vi "OFBS_test_Classifier.vi"(6 "Test Data":T2, 8 "error in (no error)":errorcluster, 9 "Classifier Session":T1, 10 "Parameters":i32[](array[numeric]), 11 "OFBS class in":refnum<class "OptFreqBandsSearch.lvclass">) -> (0 "error out":errorcluster, 1 "Confusion Matrix":i32[][](array[numeric]), 2 "Accuracy":dbl, 3 "OFBS class out":refnum<class "OptFreqBandsSearch.lvclass">)   [LabVIEW 2016, in "Optimal Frequency Bands Search.lvlib" / "OptFreqBandsSearch.lvclass"]
doc: "Метод, реализующий тестирование классификатора на основе многослойного персептрона. Для тестирования могут использоваться обучающие, либо тестовые данные"
uses:
  OptFreqBandsSearch.lvclass
  OFBS_DataTypes.ctl
  <vilib>/vision/Classification.llb/IMAQ Classifier Session.ctl
  OptFreqBandsSearch.lvclass/OptFreqBandsSearch.ctl
  4. Accuracy Assessment for EEG Classification/_vlib/CU_CohenKappa.vi
  Optimal Frequency Bands Search.lvlib
  <vilib>/addons/Machine Learning/NILabs_MLT.lvlib
  <vilib>/vision/NI_Vision_Development_Module.lvlib
  4. Accuracy Assessment for EEG Classification/Classifier.lvlib
panel:
  # "This VI is a part of BCI Design library, http://www.ru-bci.org \nCopyright © 2020, Sotnikov Peter, All rights reserved. License: GNU GPLv3"
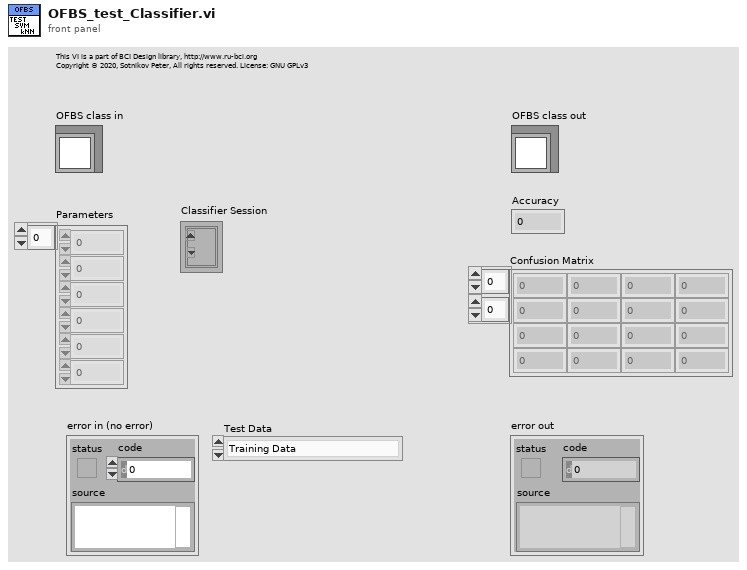
[diagram p1: front panel]
types:
  T1 = typedef "IMAQ Classifier Session.ctl" = refnum<k1>
  T2 = typedef "Optimal Frequency Bands Search.lvlib/OFBS_DataTypes.ctl" = enum16{"Training Data", "Test Data", "Training Data (cross-check)", "Test Data (cross-check)"}
  T3 = typedef "Classifier.lvlib/CU_ClassifierQualityMeasure.ctl" = enum16{"Accuracy", "Cohen's kappa"}
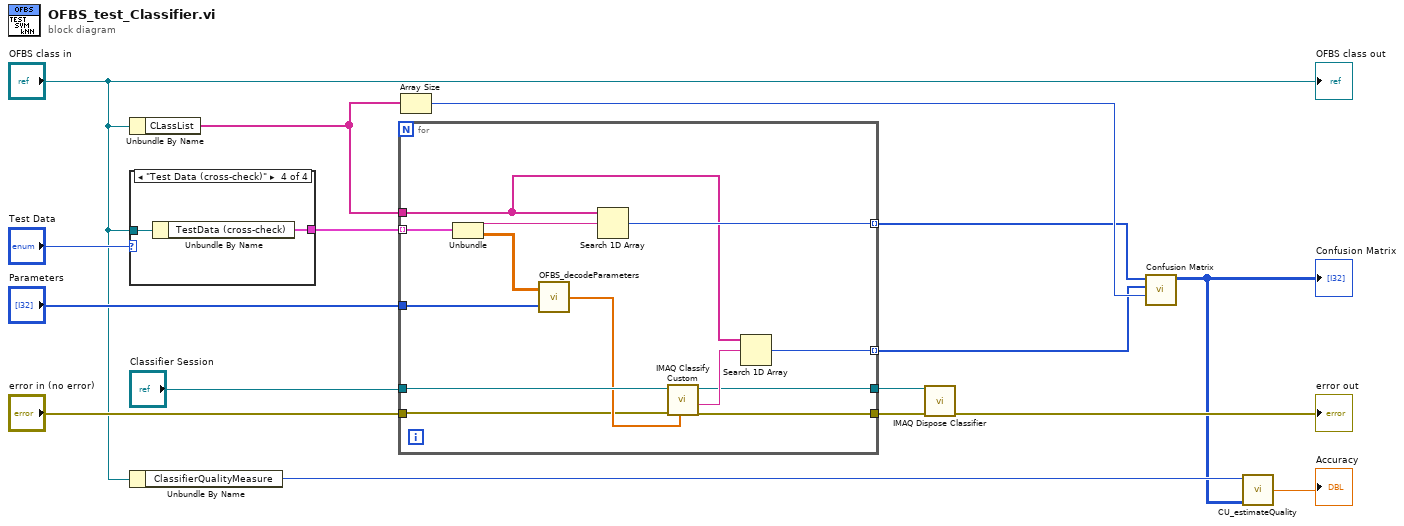
[diagram p0: block diagram]
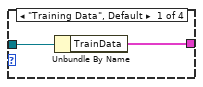
[diagram p2: hidden frame]
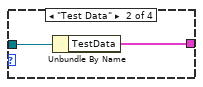
[diagram p3: hidden frame]
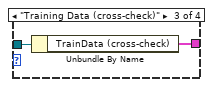
[diagram p4: hidden frame]
diagram:
  n1 = Unbundle By Name("OFBS class in") -> ("CLassList"=w12:string[])
  n2 = case shown="\"Test Data (cross-check)\"" "Test Data" {
    tunnel: "OFBS class in" -> [w18 w20 w22 w24]
    tunnel: [w17 w19 w21 w23] -> w11
    frame "Training Data", Default {
      n3 = Unbundle By Name(w18) -> ("TrainData"=w17:cluster{"ClassLabel":string, "Trial":dbl[][]}[])
    }
    frame "Test Data" {
      n4 = Unbundle By Name(w20) -> ("TestData"=w19:cluster{"ClassLabel":string, "Trial":dbl[][]}[])
    }
    frame "Training Data (cross-check)" {
      n5 = Unbundle By Name(w22) -> ("TrainData (cross-check)"=w21:cluster{"ClassLabel":string, "Trial":dbl[][]}[])
    }
    frame "Test Data (cross-check)" {
      n6 = Unbundle By Name(w24) -> ("TestData (cross-check)"=w23:cluster{"ClassLabel":string, "Trial":dbl[][]}[])
    }
  }
  n7 = Unbundle By Name("OFBS class in") -> ("ClassifierQualityMeasure"=w3:T3)
  n8 = for {
    tunnel: w11 -> [w37] mode=indexing
    tunnel: "Parameters" -> [w35]
    tunnel: w12 -> [w28]
    tunnel: [w33] -> w14 mode=indexing
    tunnel: "Classifier Session" -> [w32]
    tunnel: "error in (no error)" -> [w30]
    tunnel: [w27] -> w8
    tunnel: [w26] -> w7
    tunnel: [w25] -> w5 mode=indexing
    n9 = Unbundle(w37) -> ("ClassLabel"=w34:string, "Trial"=w36:dbl[][])
    n10 = call "OFBS_decodeParameters.vi"("Parameters"=w35, "Trial"=w36) -> ("FeatureVector"=w31:dbl[])
    n11 = Search 1D Array(1D array=w28, element=w34) -> (index of element=w33:i32)  [unwired: 1 in]
    n12 = call "IMAQ Classify Custom"("Feature Vector"=w31, "error in (no error)"=w30, "Classifier Session"=w32) -> ("error out"=w26:errorcluster, "Class"=w29:string, "Classifier Session (dup)"=w27:T1)  [unwired: 3 in, 3 out]
    n13 = Search 1D Array(1D array=w28, element=w29) -> (index of element=w25:i32)  [unwired: 1 in]
  }
  n14 = Array Size(array=w12) -> (size(s)=w15:i32)
  n15 = call "IMAQ Dispose Classifier"("error in (no error)"=w7, "Classifier Session"=w8) -> ("error out"=→"error out":errorcluster)  [unwired: 9 in]
  n16 = call <vilib>:"Confusion Matrix.vi"("# of classes"=w15, "Predicted class labels"=w5, "Actual class labels"=w14) -> ("Confusion Matrix"=w2:i32[][])  [unwired: 7 in, 1 out]
  "Confusion Matrix" <- w2
  n17 = call "CU_estimateQuality.vi"("Quality Measure in"=w3, "Confusion Matrix in"=w2) -> ("Classification Quality out"=→"Accuracy":dbl)  [unwired: 6 in]
  "OFBS class out" <- "OFBS class in"
